vi "启动参数设置.vi"() -> ()   [LabVIEW 2016, in "斯坦道总氮.lvlib"]
panel:
  in  "保存":bool
  out "启动队列名称":cluster{"String":string, "Value":u16}[](array[cluster])
  out "启动参数":string
  in  "CODCr":bool
  in  "硫化物":bool
  in  "硅酸盐":bool
  in  "亚硝氮":bool
  in  "硝氮":bool
  in  "磷酸盐":bool
  in  "氨氮":bool
  in  "总氮":bool
  in  "总磷":bool
  # "请选择要启动的参数"
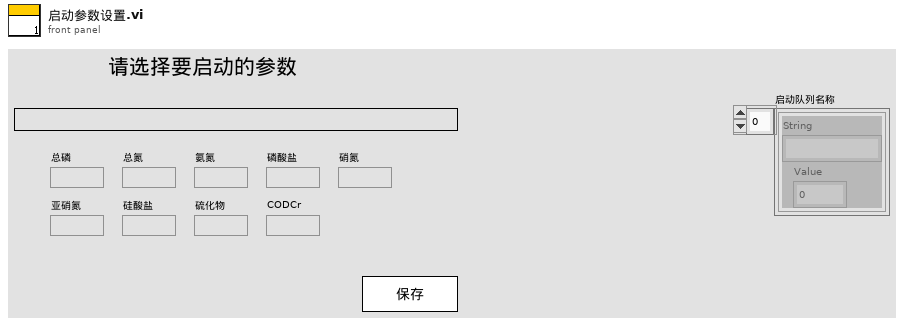
[diagram p1: front panel]
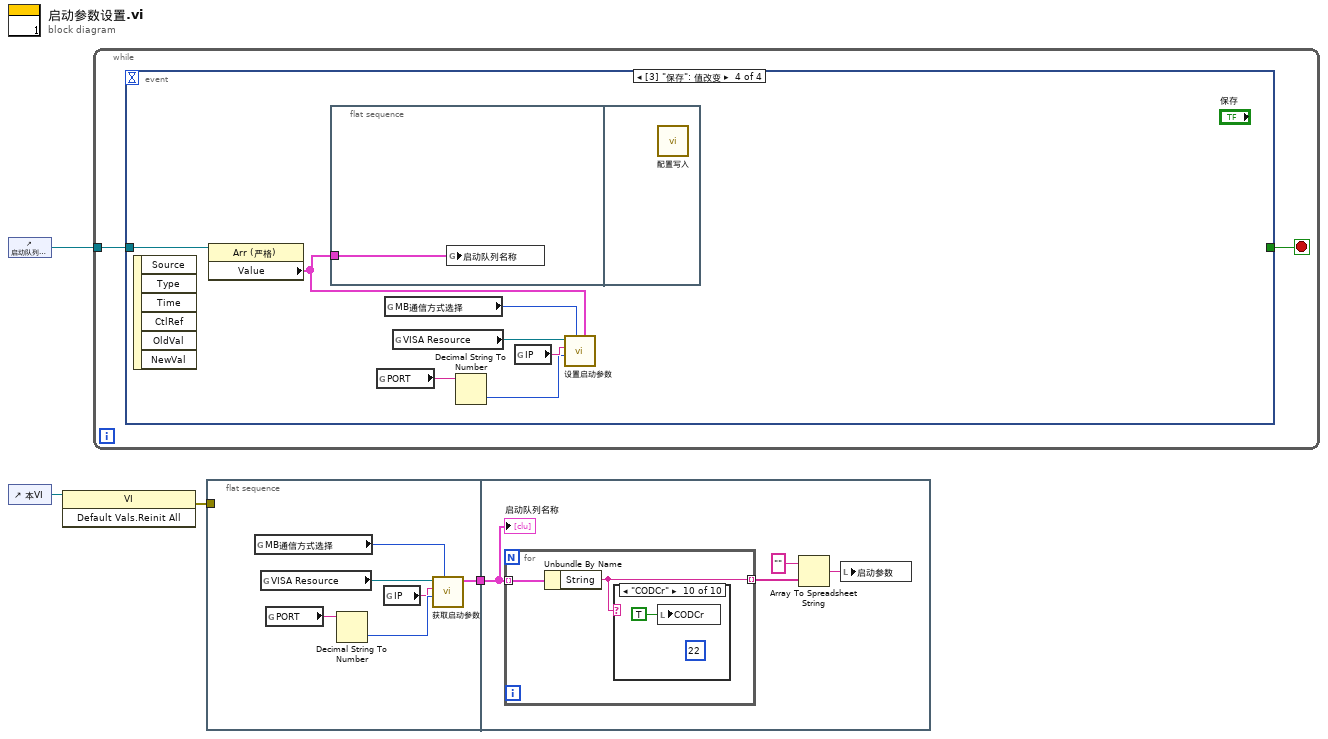
[diagram p0: block diagram]
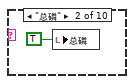
[diagram p3: hidden frame]
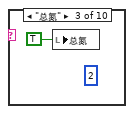
[diagram p4: hidden frame]
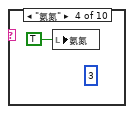
[diagram p5: hidden frame]
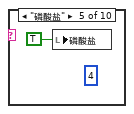
[diagram p6: hidden frame]
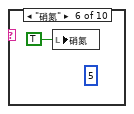
[diagram p7: hidden frame]
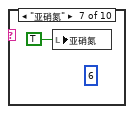
[diagram p8: hidden frame]
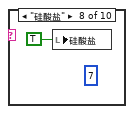
[diagram p9: hidden frame]
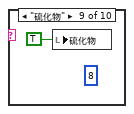
[diagram p10: hidden frame]
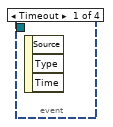
[diagram p11: hidden frame]
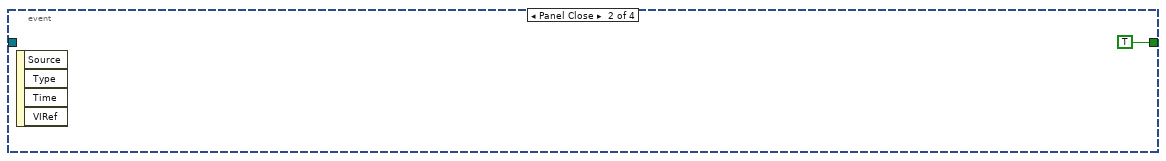
[diagram p12: hidden frame]
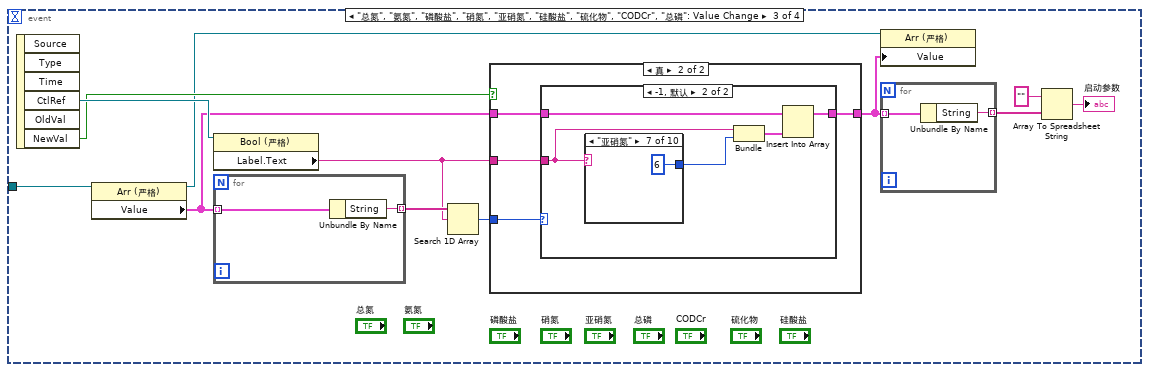
[diagram p13: hidden frame]
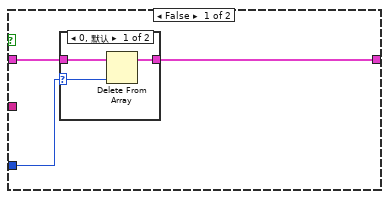
[diagram p14: hidden frame]
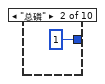
[diagram p18: hidden frame]
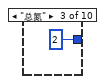
[diagram p19: hidden frame]
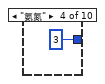
[diagram p20: hidden frame]
diagram:
  n1 = control-ref of="启动队列名称"() -> (w4:refnum<vi>)
  n2 = control-ref of="本VI"() -> (w3:refnum<vi>)
  n3 = invoke class="VI" method="Default Vals.Reinit All"(reference=w3) -> (error out=w2:errorcluster)  [unwired: 2 in, 2 out]
  n4 = while {
    tunnel: w4 -> [w5]
    stop <- w6 stop-if-true
    n5 = event shown="[3] \"保存\": 值改变" {
      selector: _ -> [_ _ _ _]
      dyn-events: _ -> [_ _ _ _]
      timeout: _ -> [_ _ _ _]
      tunnel: [_ TRUE _ _] -> w6
      tunnel: w5 -> [_ _ w11 w56]
      event Timeout {
        n6 = event-data() -> ()  [unwired: 1 in, 3 out]
      }
      event Panel Close {
        n7 = event-data() -> ()  [unwired: 1 in, 4 out]
      }
      event "总氮", "氨氮", "磷酸盐", "硝氮", "亚硝氮", "硅酸盐", "硫化物", "CODCr", "总磷": Value Change {
        n8 = event-data() -> ("CtlRef"=w19:refnum<vi>, "NewVal"=w18:bool)  [unwired: 1 in, 4 out]
        n9 = property class="Arr (严格)"(reference=w11) -> (reference out=w9:refnum<vi>, "Value"=w10:cluster{"String":string, "Value":u16}[])  [unwired: 1 in, 1 out]
        n10 = property class="Bool (严格)"(reference=w19) -> ("Label.Text"=w16:string)  [unwired: 1 in, 2 out]
        n11 = for {
          tunnel: w10 -> [w23] mode=indexing
          tunnel: [w22] -> w17 mode=indexing
          n12 = Unbundle By Name(w23) -> ("String"=w22:string)
        }
        n13 = Search 1D Array(1D array=w17, element=w16) -> (index of element=w15:i32)  [unwired: 1 in]
        n14 = case shown="真" w18 {
          tunnel: w16 -> [_ w33]
          tunnel: w10 -> [w25 w34]
          tunnel: w15 -> [w26 w32]
          tunnel: [w24 w31] -> w8
          frame False {
            n15 = case shown="0, 默认" w26 {
              selector: w26 -> [w28 _]
              tunnel: w25 -> [w29 w30]
              tunnel: [w27 w30] -> w24
              frame 0, Default {
                n16 = Delete From Array(array=w29, index=w28) -> (array with subset deleted=w27:cluster{"String":string, "Value":u16}[])  [unwired: 1 in, 1 out]
              }
              frame -1 {
              }
            }
          }
          frame True {
            n17 = case shown="-1, 默认" w32 {
              tunnel: w34 -> [w35 w40]
              tunnel: w33 -> [_ w39]
              tunnel: [w35 w36] -> w31
              frame 0 {
              }
              frame -1, Default {
                n18 = case shown="\"亚硝氮\"" w39 {
                  tunnel: [_ 1 2 3 4 5 6 7 8 22] -> w38
                  frame Default {
                  }
                  frame "总磷" {
                  }
                  frame "总氮" {
                  }
                  frame "氨氮" {
                  }
                  frame "磷酸盐" {
                  }
                  frame "硝氮" {
                  }
                  frame "亚硝氮" {
                  }
                  frame "硅酸盐" {
                  }
                  frame "硫化物" {
                  }
                  frame "CODCr" {
                  }
                }
                n19 = Bundle("Label.Text"=w39, w38) -> (w37:cluster{"Label.Text":string, i32})  [unwired: 1 in]
                n20 = Insert Into Array(array=w40, new element=w37) -> (w36:cluster{"String":string, "Value":u16}[])  [unwired: 1 in]
              }
            }
          }
        }
        n21 = property class="Arr (严格)"(reference=w9, "Value"=w8) -> ()  [unwired: 1 in, 2 out]
        n22 = for {
          tunnel: w8 -> [w21] mode=indexing
          tunnel: [w20] -> w14 mode=indexing
          n23 = Unbundle By Name(w21) -> ("String"=w20:string)
        }
        n24 = Array To Spreadsheet String(array=w14, 3:"" ("格式字符串")) -> (spreadsheet string=→"启动参数":string)  [unwired: 1 in]
      }
      event "保存": Value Change {
        n25 = event-data() -> ()  [unwired: 1 in, 6 out]
        n26 = property class="Arr (严格)"(reference=w56) -> ("Value"=w50:cluster{"String":string, "Value":u16}[])  [unwired: 1 in, 2 out]
        n27 = flat-sequence {
          tunnel: w50 -> [w57]
          frame #0 {
            n28 = global write "总磷总氮断电保存全局变量.vi" "启动队列名称"(w57) -> ()
          }
          frame #1 {
            n29 = call "配置写入.vi"() -> ()  [unwired: 11 in, 1 out]
          }
        }
        n30 = global read "总磷总氮断电保存全局变量.vi" "PORT"() -> (w52:string)
        n31 = global read "总磷总氮断电保存全局变量.vi" "MB通信方式选择"() -> (w55:enum16{"串口", "TCP"})
        n32 = global read "总磷总氮断电保存全局变量.vi" "VISA Resource"() -> (w54:refnum<visa-resource-name>)
        n33 = Decimal String To Number(string=w52) -> (number=w51:i32)  [unwired: 2 in, 1 out]
        n34 = global read "总磷总氮断电保存全局变量.vi" "IP"() -> (w53:string)
        n35 = call "设置启动参数.vi"("数组"=w50, "MB通信方式选择"=w55, "Port (502)"=w51, "IP Address"=w53, "VISA Resource"=w54) -> ()  [unwired: 6 in, 1 out]
      }
    }
  }
  n36 = flat-sequence {
    tunnel: w2 -> [_]
    tunnel: [w58] -> w1
    tunnel: w1 -> [w64]
    frame #0 {
      n37 = global read "总磷总氮断电保存全局变量.vi" "MB通信方式选择"() -> (w60:enum16{"串口", "TCP"})
      n38 = global read "总磷总氮断电保存全局变量.vi" "VISA Resource"() -> (w61:refnum<visa-resource-name>)
      n39 = global read "总磷总氮断电保存全局变量.vi" "PORT"() -> (w59:string)
      n40 = Decimal String To Number(string=w59) -> (number=w63:i32)  [unwired: 2 in, 1 out]
      n41 = global read "总磷总氮断电保存全局变量.vi" "IP"() -> (w62:string)
      n42 = call "获取启动参数.vi"("MB通信方式选择"=w60, "Port (502)"=w63, "IP Address"=w62, "VISA Resource"=w61) -> ("数组"=w58:cluster{"String":string, "Value":u16}[])  [unwired: 6 in, 1 out]
    }
    frame #1 {
      n43 = for {
        tunnel: w64 -> [w69] mode=indexing
        tunnel: [w68] -> w66 mode=indexing
        n44 = Unbundle By Name(w69) -> ("String"=w68:string)
        n45 = case shown="\"CODCr\"" w68 {
          frame Default {
          }
          frame "总磷" {
            n46 = local write "总磷"(TRUE ("总磷")) -> ()
          }
          frame "总氮" {
            (unwired) 2
            n47 = local write "总氮"(TRUE ("总磷")) -> ()
          }
          frame "氨氮" {
            (unwired) 3
            n48 = local write "氨氮"(TRUE ("总磷")) -> ()
          }
          frame "磷酸盐" {
            (unwired) 4
            n49 = local write "磷酸盐"(TRUE ("总磷")) -> ()
          }
          frame "硝氮" {
            (unwired) 5
            n50 = local write "硝氮"(TRUE ("总磷")) -> ()
          }
          frame "亚硝氮" {
            (unwired) 6
            n51 = local write "亚硝氮"(TRUE ("总磷")) -> ()
          }
          frame "硅酸盐" {
            (unwired) 7
            n52 = local write "硅酸盐"(TRUE ("总磷")) -> ()
          }
          frame "硫化物" {
            (unwired) 8
            n53 = local write "硫化物"(TRUE ("总磷")) -> ()
          }
          frame "CODCr" {
            (unwired) 22
            n54 = local write "CODCr"(TRUE ("总磷")) -> ()
          }
        }
      }
      n55 = Array To Spreadsheet String(array=w66, 3:"" ("格式字符串")) -> (spreadsheet string=w65:string)  [unwired: 1 in]
      n56 = local write "启动参数"(w65) -> ()
      "启动队列名称" <- w64
    }
  }
